vi "Arm State Controller.vi"() -> ()   [LabVIEW 2020]
uses:
  <vilib>/Rock Robotics/WPI/ThirdParty/REV Robotics/REVLib/Typedef/Spark MAX Control Type.ctl
panel:
  out "Completed Arm State":T1(ring)
  in  "Last Manual Shoulder State":dbl
  in  "Last Manual Elbow State":dbl
  in  "Target Arm State":T1(ring)
  in  "Previous Arm State":T2(ring)
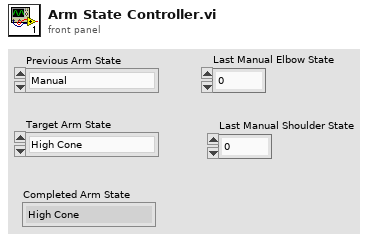
[diagram p1: front panel]
types:
  T1 = enum16{"High Cone", "Manual", "High Cube", "Mid Cone", "Mid Cube", "Intake", "Cube Handoff", "Cone Handoff", "Stow"}
  T2 = enum16{"Manual", "High Cone", "High Cube", "Mid Cone", "Mid Cube", "Intake", "Cube Handoff", "Cone Handoff", "Stow"}
  T3 = cluster{"Stow Shoulder Setpoint":dbl, "Intake Shoulder Setpoint":dbl, "Cube Handoff Shoulder Setpoint":dbl, "Cone Handoff Shoulder Setpoint":dbl, "Mid Cone Shoulder Setpoint":dbl, "Mid Cube Shoulder Setpoint":dbl, "High Cone Shoulder Setpoint":dbl, "High Cube Shoulder Setpoint":dbl}
  T4 = cluster{"Stow Elbow Setpoint":dbl, "Intake Elbow Setpoint":dbl, "Cube Handoff Elbow Setpoint":dbl, "Cone Handoff Elbow Setpoint":dbl, "Mid Cone Elbow Setpoint":dbl, "Mid Cube Elbow Setpoint":dbl, "High Cone Elbow Setpoint":dbl, "High Cube Elbow Setpoint":dbl}
  T5 = enum16{"To Manual", "From Manual", "Motion Profile", "PID Only"}
  T6 = typedef "Spark MAX Control Type.ctl" = enum16{"Percent VBus", "Voltage", "Velocity", "Position", "Smart Motion", "Current", "Smart Velocity"}
  T7 = typedef "WPI_MotorControlDeviceRef.ctl" = cluster{"DeviceStatus":errorcluster, "Type":T8, "PWM":cluster{"PWM Channel":T9, "DeadBand":T10}, "CAN":cluster{"Device Number":u8, "SetOutput VI Ref":variant, "GetOutput VI Ref":variant, "Enable VI Ref":variant, "Disable VI Ref":variant, "Data":variant}, "Invert":bool, "DIO PWM":cluster{"PWM \"Enable\" Channel":T9, "DIOChannel":T11, "PWM Rate":dbl}}
  T8 = typedef "WPI_MotorControlType.ctl" = enum16{"PWM", "CAN", "DIO PWM"}
  T9 = typedef "FPGA_DIOPWMChannel.ctl" = enum8{"PWM 0", "PWM 1", "PWM 2", "PWM 3", "PWM 4", "PWM 5", "PWM 6", "PWM 7", "PWM 8", "PWM 9", "PWM MXP 0", "PWM MXP 1", "PWM MXP 2", "PWM MXP 3", "PWM MXP 4", "PWM MXP 5", "PWM MXP 6", "PWM MXP 7", "PWM MXP 8", "PWM MXP 9", "Invalid"}
  T10 = typedef "WPI_PWMDeadband.ctl" = cluster{"Name":string, "maxPositivePwm":i32, "minPositivePwm":i32, "centerPwm":i32, "maxNegativePwm":i32, "minNegativePwm":i32, "angularRange":u16}
  T11 = typedef "FPGA_DIOChannel.ctl" = enum8{"DIO 0", "DIO 1", "DIO 2", "DIO 3", "DIO 4", "DIO 5", "DIO 6", "DIO 7", "DIO 8", "DIO 9", "DIO MXP 0", "DIO MXP 1", "DIO MXP 2", "DIO MXP 3", "DIO MXP 4", "DIO MXP 5", "DIO MXP 6", "DIO MXP 7", "DIO MXP 8", "DIO MXP 9", "DIO MXP 10", "DIO MXP 11", "DIO MXP 12", "DIO MXP 13", "DIO MXP 14", "DIO MXP 15", "SPI Port CS1", "SPI Port CS2", "SPI Port CS3", "SPI Port MISO", "SPI Port MOSI", "Invalid"}
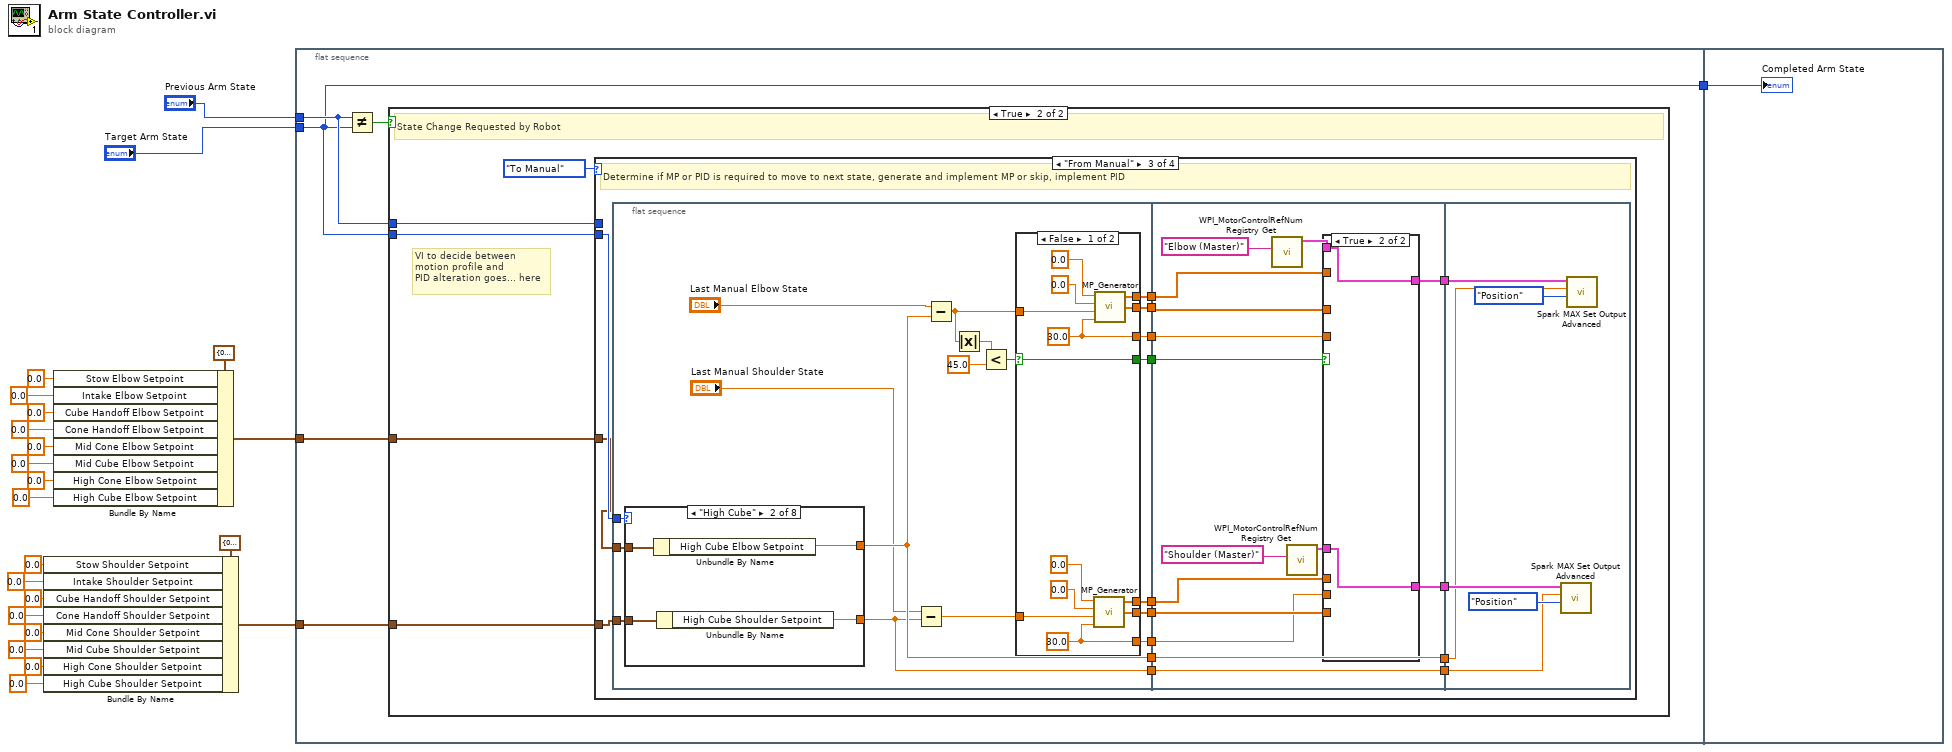
[diagram p0: block diagram]
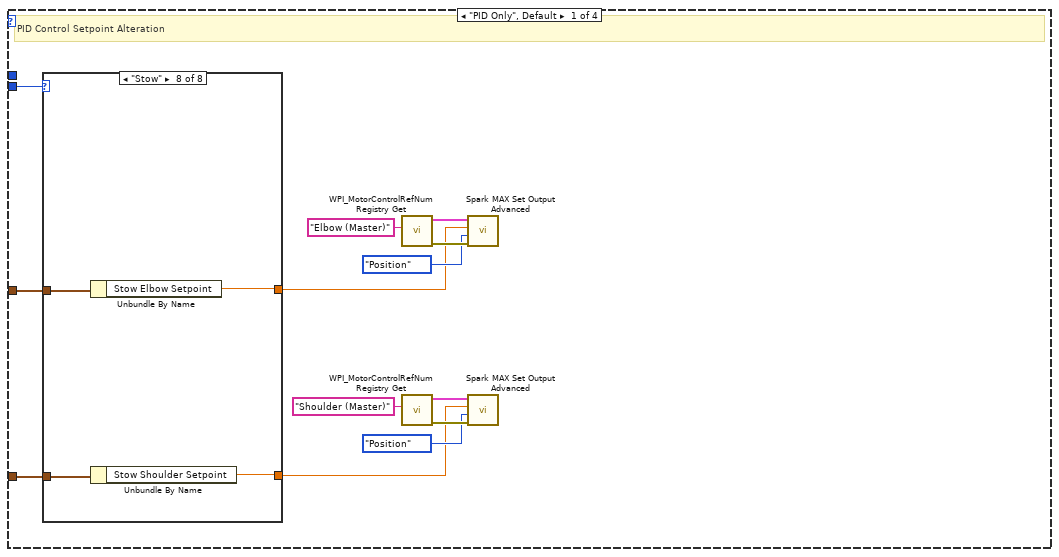
[diagram p3: hidden frame]
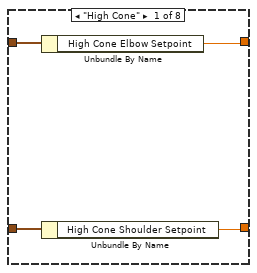
[diagram p4: hidden frame]
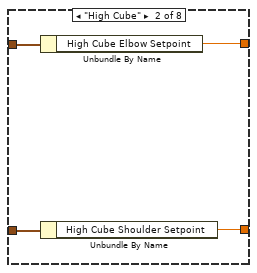
[diagram p5: hidden frame]
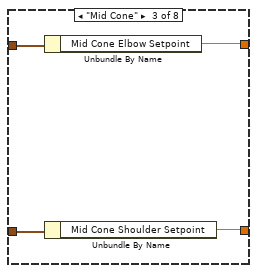
[diagram p6: hidden frame]
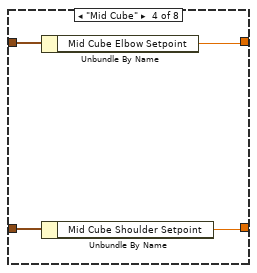
[diagram p7: hidden frame]
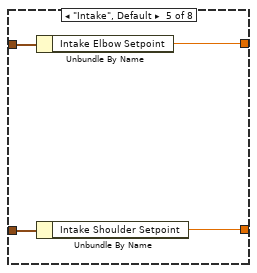
[diagram p8: hidden frame]
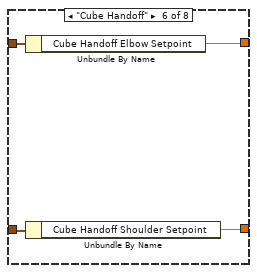
[diagram p9: hidden frame]
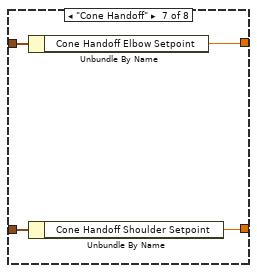
[diagram p10: hidden frame]
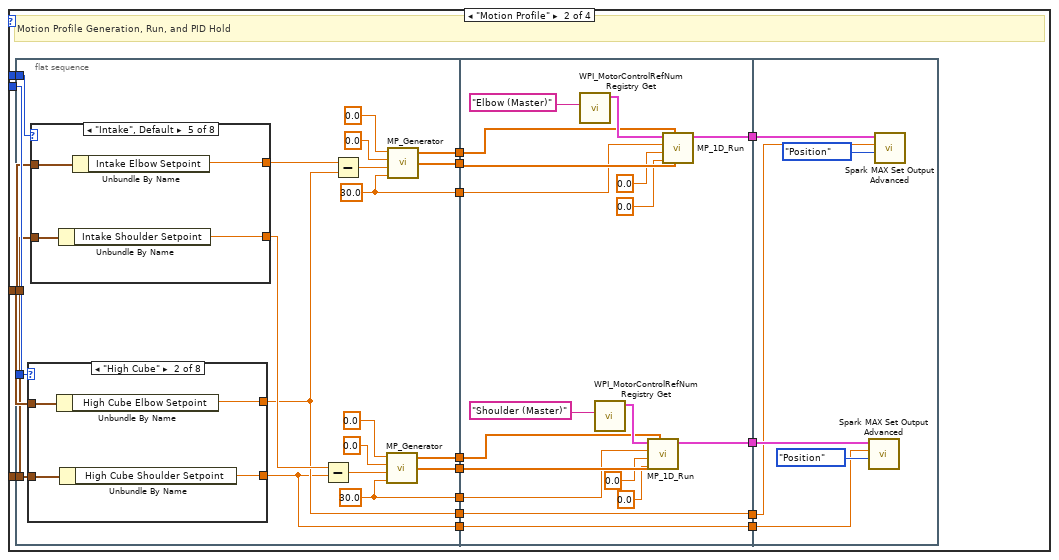
[diagram p11: hidden frame]
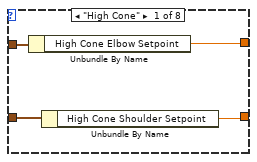
[diagram p12: hidden frame]
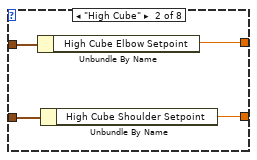
[diagram p13: hidden frame]
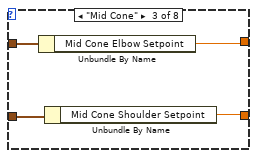
[diagram p14: hidden frame]
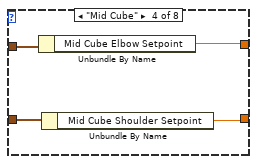
[diagram p15: hidden frame]
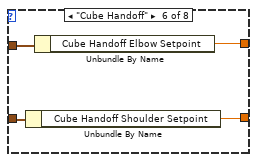
[diagram p16: hidden frame]
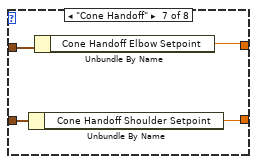
[diagram p17: hidden frame]
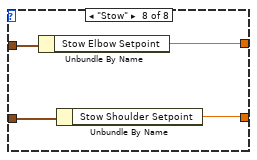
[diagram p18: hidden frame]
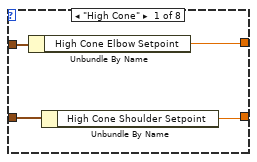
[diagram p19: hidden frame]
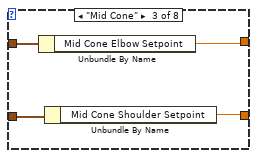
[diagram p20: hidden frame]
diagram:
  n1 = Bundle By Name(cluster=T3 {"Stow Shoulder Setpoint"=0.0, "Intake Shoulder Setpoint"=0.0, "Cube Handoff Shoulder Setpoint"=0.0, "Cone Handoff Shoulder Setpoint"=0.0, "Mid Cone Shoulder Setpoint"=0.0, "Mid Cube Shoulder Setpoint"=0.0, "High Cone Shoulder Setpoint"=0.0, "High Cube Shoulder Setpoint"=0.0}, "Stow Shoulder Setpoint"=0.0 ("Stow Elbow Setpoint"), "Intake Shoulder Setpoint"=0.0 ("Intake Elbow Setpoint"), "Cube Handoff Shoulder Setpoint"=0.0 ("Cube Handoff Elbow Setpoint"), "Cone Handoff Shoulder Setpoint"=0.0 ("Cone Handoff Elbow Setpoint"), "Mid Cone Shoulder Setpoint"=0.0 ("Mid Cone Elbow Setpoint"), "Mid Cube Shoulder Setpoint"=0.0 ("Mid Cube Elbow Setpoint"), "High Cone Shoulder Setpoint"=0.0 ("High Cone Elbow Setpoint"), "High Cube Shoulder Setpoint"=0.0 ("High Cube Elbow Setpoint")) -> (w4:T3)
  n2 = Bundle By Name(cluster=T4 {"Stow Elbow Setpoint"=0.0, "Intake Elbow Setpoint"=0.0, "Cube Handoff Elbow Setpoint"=0.0, "Cone Handoff Elbow Setpoint"=0.0, "Mid Cone Elbow Setpoint"=0.0, "Mid Cube Elbow Setpoint"=0.0, "High Cone Elbow Setpoint"=0.0, "High Cube Elbow Setpoint"=0.0}, "Stow Elbow Setpoint"=0.0, "Intake Elbow Setpoint"=0.0, "Cube Handoff Elbow Setpoint"=0.0, "Cone Handoff Elbow Setpoint"=0.0, "Mid Cone Elbow Setpoint"=0.0, "Mid Cube Elbow Setpoint"=0.0, "High Cone Elbow Setpoint"=0.0, "High Cube Elbow Setpoint"=0.0) -> (w5:T4)
  n3 = flat-sequence {
    tunnel: w5 -> [w27]
    tunnel: w4 -> [w26]
    tunnel: "Target Arm State" -> [w24]
    tunnel: "Previous Arm State" -> [w25]
    tunnel: [w24] -> w1
    tunnel: w1 -> [w324]
    frame #0 {
      n4 = Not Equal?(x=w25, y=w24) -> (x != y?=w28:bool)
      n5 = case shown="True" w28 {
        tunnel: w27 -> [_ w31]
        tunnel: w26 -> [_ w33]
        tunnel: w24 -> [_ w32]
        tunnel: w25 -> [_ w30]
        frame False {
          # "No State Change Detected"
        }
        frame True {
          # "VI to decide between\nmotion profile and \nPID alteration goes... here"
          # "State Change Requested by Robot"
          n6 = case shown="\"From Manual\"" T5."To Manual" {
            tunnel: w33 -> [w42 w92 w205 _]
            tunnel: w32 -> [w41 w94 w206 _]
            tunnel: w31 -> [w39 w93 w204 _]
            tunnel: w30 -> [_ w91 _ _]
            frame "PID Only", Default {
              # "PID Control Setpoint Alteration"
              n7 = case shown="\"Stow\"" w41 {
                tunnel: w42 -> [w48 w52 w56 w60 w66 w67 w71 w76]
                tunnel: [w47 w51 w55 w59 w65 w68 w72 w75] -> w40
                tunnel: w39 -> [w50 w54 w58 w62 w64 w70 w74 w78]
                tunnel: [w49 w53 w57 w61 w63 w69 w73 w77] -> w34
                frame "High Cone" {
                  n8 = Unbundle By Name(w50) -> ("High Cone Elbow Setpoint"=w49:dbl)
                  n9 = Unbundle By Name(w48) -> ("High Cone Shoulder Setpoint"=w47:dbl)
                }
                frame "High Cube" {
                  n10 = Unbundle By Name(w54) -> ("High Cube Elbow Setpoint"=w53:dbl)
                  n11 = Unbundle By Name(w52) -> ("High Cube Shoulder Setpoint"=w51:dbl)
                }
                frame "Mid Cone" {
                  n12 = Unbundle By Name(w58) -> ("Mid Cone Elbow Setpoint"=w57:dbl)
                  n13 = Unbundle By Name(w56) -> ("Mid Cone Shoulder Setpoint"=w55:dbl)
                }
                frame "Mid Cube" {
                  n14 = Unbundle By Name(w62) -> ("Mid Cube Elbow Setpoint"=w61:dbl)
                  n15 = Unbundle By Name(w60) -> ("Mid Cube Shoulder Setpoint"=w59:dbl)
                }
                frame "Intake", Default {
                  n16 = Unbundle By Name(w64) -> ("Intake Elbow Setpoint"=w63:dbl)
                  n17 = Unbundle By Name(w66) -> ("Intake Shoulder Setpoint"=w65:dbl)
                }
                frame "Cube Handoff" {
                  n18 = Unbundle By Name(w70) -> ("Cube Handoff Elbow Setpoint"=w69:dbl)
                  n19 = Unbundle By Name(w67) -> ("Cube Handoff Shoulder Setpoint"=w68:dbl)
                }
                frame "Cone Handoff" {
                  n20 = Unbundle By Name(w74) -> ("Cone Handoff Elbow Setpoint"=w73:dbl)
                  n21 = Unbundle By Name(w71) -> ("Cone Handoff Shoulder Setpoint"=w72:dbl)
                }
                frame "Stow" {
                  n22 = Unbundle By Name(w78) -> ("Stow Elbow Setpoint"=w77:dbl)
                  n23 = Unbundle By Name(w76) -> ("Stow Shoulder Setpoint"=w75:dbl)
                }
              }
              n24 = call <vilib>:"WPI_MotorControlRefNum Registry Get.vi"("refnum name"="Elbow (Master)") -> ("error out"=w36:errorcluster, "MotorControlDevRef"=w37:T7)  [unwired: 9 in]
              n25 = call <vilib>:"WPI_MotorControlRefNum Registry Get.vi"("refnum name"="Shoulder (Master)") -> ("error out"=w44:errorcluster, "MotorControlDevRef"=w45:T7)  [unwired: 9 in]
              n26 = call <vilib>:"Spark MAX Set Output Advanced.vi"("error in (no error)"=w36, "Control Mode"=Spark_MAX_Control_Type."Position", "Setpoint"=w34, "MotorControlDevRef"=w37) -> ()  [unwired: 6 in, 2 out]
              n27 = call <vilib>:"Spark MAX Set Output Advanced.vi"("error in (no error)"=w44, "Control Mode"=Spark_MAX_Control_Type."Position", "Setpoint"=w40, "MotorControlDevRef"=w45) -> ()  [unwired: 6 in, 2 out]
            }
            frame "Motion Profile" {
              # "Motion Profile Generation, Run, and PID Hold"
              n28 = flat-sequence {
                tunnel: w94 -> [w114]
                tunnel: w93 -> [w113]
                tunnel: w92 -> [w112]
                tunnel: w91 -> [w111]
                tunnel: [w106] -> w90
                tunnel: [w105] -> w89
                tunnel: [w100] -> w88
                tunnel: [w99] -> w87
                tunnel: [w98] -> w83
                tunnel: [w97] -> w82
                tunnel: [w96] -> w80
                tunnel: [w95] -> w79
                tunnel: w90 -> [w190]
                tunnel: w89 -> [w189]
                tunnel: w88 -> [w183]
                tunnel: w87 -> [w182]
                tunnel: [w185] -> w86
                tunnel: [w192] -> w85
                tunnel: [w194] -> w84
                tunnel: w83 -> [w194]
                tunnel: w82 -> [w193]
                tunnel: [w193] -> w81
                tunnel: w80 -> [w188]
                tunnel: w79 -> [w181]
                tunnel: w86 -> [w199]
                tunnel: w85 -> [w202]
                tunnel: w84 -> [w198]
                tunnel: w81 -> [w197]
                frame #0 {
                  w95 = 30.0 ("Time Resolution (ms)")
                  w96 = 30.0 ("Time Resolution (ms)")
                  n29 = case shown="\"High Cube\"" w114 {
                    tunnel: w112 -> [w148 w152 w156 w160 w166 w167 w171 w176]
                    tunnel: [w147 w151 w155 w159 w165 w168 w172 w175] -> w97
                    tunnel: w113 -> [w150 w154 w158 w162 w164 w170 w174 w178]
                    tunnel: [w149 w153 w157 w161 w163 w169 w173 w177] -> w98
                    frame "High Cone" {
                      n30 = Unbundle By Name(w150) -> ("High Cone Elbow Setpoint"=w149:dbl)
                      n31 = Unbundle By Name(w148) -> ("High Cone Shoulder Setpoint"=w147:dbl)
                    }
                    frame "High Cube" {
                      n32 = Unbundle By Name(w154) -> ("High Cube Elbow Setpoint"=w153:dbl)
                      n33 = Unbundle By Name(w152) -> ("High Cube Shoulder Setpoint"=w151:dbl)
                    }
                    frame "Mid Cone" {
                      n34 = Unbundle By Name(w158) -> ("Mid Cone Elbow Setpoint"=w157:dbl)
                      n35 = Unbundle By Name(w156) -> ("Mid Cone Shoulder Setpoint"=w155:dbl)
                    }
                    frame "Mid Cube" {
                      n36 = Unbundle By Name(w162) -> ("Mid Cube Elbow Setpoint"=w161:dbl)
                      n37 = Unbundle By Name(w160) -> ("Mid Cube Shoulder Setpoint"=w159:dbl)
                    }
                    frame "Intake", Default {
                      n38 = Unbundle By Name(w166) -> ("Intake Shoulder Setpoint"=w165:dbl)
                      n39 = Unbundle By Name(w164) -> ("Intake Elbow Setpoint"=w163:dbl)
                    }
                    frame "Cube Handoff" {
                      n40 = Unbundle By Name(w167) -> ("Cube Handoff Shoulder Setpoint"=w168:dbl)
                      n41 = Unbundle By Name(w170) -> ("Cube Handoff Elbow Setpoint"=w169:dbl)
                    }
                    frame "Cone Handoff" {
                      n42 = Unbundle By Name(w171) -> ("Cone Handoff Shoulder Setpoint"=w172:dbl)
                      n43 = Unbundle By Name(w174) -> ("Cone Handoff Elbow Setpoint"=w173:dbl)
                    }
                    frame "Stow" {
                      n44 = Unbundle By Name(w178) -> ("Stow Elbow Setpoint"=w177:dbl)
                      n45 = Unbundle By Name(w176) -> ("Stow Shoulder Setpoint"=w175:dbl)
                    }
                  }
                  n46 = case shown="\"Intake\", Default" w111 {
                    tunnel: w112 -> [w116 w120 w124 w128 w134 w135 w139 w144]
                    tunnel: [w115 w119 w123 w127 w133 w136 w140 w143] -> w104
                    tunnel: w113 -> [w118 w122 w126 w130 w132 w138 w142 w146]
                    tunnel: [w117 w121 w125 w129 w131 w137 w141 w145] -> w110
                    frame "High Cone" {
                      n47 = Unbundle By Name(w118) -> ("High Cone Elbow Setpoint"=w117:dbl)
                      n48 = Unbundle By Name(w116) -> ("High Cone Shoulder Setpoint"=w115:dbl)
                    }
                    frame "High Cube" {
                      n49 = Unbundle By Name(w122) -> ("High Cube Elbow Setpoint"=w121:dbl)
                      n50 = Unbundle By Name(w120) -> ("High Cube Shoulder Setpoint"=w119:dbl)
                    }
                    frame "Mid Cone" {
                      n51 = Unbundle By Name(w126) -> ("Mid Cone Elbow Setpoint"=w125:dbl)
                      n52 = Unbundle By Name(w124) -> ("Mid Cone Shoulder Setpoint"=w123:dbl)
                    }
                    frame "Mid Cube" {
                      n53 = Unbundle By Name(w130) -> ("Mid Cube Elbow Setpoint"=w129:dbl)
                      n54 = Unbundle By Name(w128) -> ("Mid Cube Shoulder Setpoint"=w127:dbl)
                    }
                    frame "Intake", Default {
                      n55 = Unbundle By Name(w134) -> ("Intake Shoulder Setpoint"=w133:dbl)
                      n56 = Unbundle By Name(w132) -> ("Intake Elbow Setpoint"=w131:dbl)
                    }
                    frame "Cube Handoff" {
                      n57 = Unbundle By Name(w135) -> ("Cube Handoff Shoulder Setpoint"=w136:dbl)
                      n58 = Unbundle By Name(w138) -> ("Cube Handoff Elbow Setpoint"=w137:dbl)
                    }
                    frame "Cone Handoff" {
                      n59 = Unbundle By Name(w139) -> ("Cone Handoff Shoulder Setpoint"=w140:dbl)
                      n60 = Unbundle By Name(w142) -> ("Cone Handoff Elbow Setpoint"=w141:dbl)
                    }
                    frame "Stow" {
                      n61 = Unbundle By Name(w146) -> ("Stow Elbow Setpoint"=w145:dbl)
                      n62 = Unbundle By Name(w144) -> ("Stow Shoulder Setpoint"=w143:dbl)
                    }
                  }
                  n63 = Subtract(x=w104, y=w97) -> (x-y=w101:dbl)
                  n64 = Subtract(x=w110, y=w98) -> (x-y=w109:dbl)
                  n65 = call "MP_Generator.vi"("Time Resolution (ms)"=w95, "Goal (deg)"=w101, "Maximum Acceleration (deg/s^2)"=0.0, "Maximum Velocity (deg/s)"=0.0) -> ("Timestamp (s)"=w99:dbl[], "Velocity (deg/s)"=w100:dbl[])  [unwired: 1 out]
                  n66 = call "MP_Generator.vi"("Time Resolution (ms)"=w96, "Goal (deg)"=w109, "Maximum Acceleration (deg/s^2)"=0.0, "Maximum Velocity (deg/s)"=0.0) -> ("Timestamp (s)"=w105:dbl[], "Velocity (deg/s)"=w106:dbl[])  [unwired: 1 out]
                }
                frame #1 {
                  n67 = call <vilib>:"WPI_MotorControlRefNum Registry Get.vi"("refnum name"="Elbow (Master)") -> ("MotorControlDevRef"=w191:T7)  [unwired: 9 in, 1 out]
                  n68 = call <vilib>:"WPI_MotorControlRefNum Registry Get.vi"("refnum name"="Shoulder (Master)") -> ("MotorControlDevRef"=w184:T7)  [unwired: 9 in, 1 out]
                  n69 = call "MP_1D_Run.vi"("Time Index"=w182, "Velocity"=w183, "Max Velocity"=0.0, "Max Acceleration"=0.0, "Time Resolution (ms)"=w181, "MotorControlDeviceRef"=w184) -> ("MotorControlDevRef"=w185:T7)  [unwired: 5 in]
                  n70 = call "MP_1D_Run.vi"("Time Index"=w189, "Velocity"=w190, "Max Velocity"=0.0, "Max Acceleration"=0.0, "Time Resolution (ms)"=w188, "MotorControlDeviceRef"=w191) -> ("MotorControlDevRef"=w192:T7)  [unwired: 5 in]
                }
                frame #2 {
                  n71 = call <vilib>:"Spark MAX Set Output Advanced.vi"("Control Mode"=Spark_MAX_Control_Type."Position", "Setpoint"=w197, "MotorControlDevRef"=w199) -> ()  [unwired: 7 in, 2 out]
                  n72 = call <vilib>:"Spark MAX Set Output Advanced.vi"("Control Mode"=Spark_MAX_Control_Type."Position", "Setpoint"=w198, "MotorControlDevRef"=w202) -> ()  [unwired: 7 in, 2 out]
                }
              }
            }
            frame "From Manual" {
              # "Determine if MP or PID is required to move to next state, generate and implement MP or skip, implement PID"
              n73 = flat-sequence {
                tunnel: w205 -> [w237]
                tunnel: [w236] -> w218
                tunnel: [w235] -> w217
                tunnel: [w234] -> w216
                tunnel: [w233] -> w215
                tunnel: [w232] -> w214
                tunnel: [w227] -> w213
                tunnel: [w231] -> w212
                tunnel: [w230] -> w211
                tunnel: w206 -> [w229]
                tunnel: w204 -> [w228]
                tunnel: [w219] -> w203
                tunnel: w218 -> [w295]
                tunnel: w217 -> [w294]
                tunnel: w216 -> [w290]
                tunnel: w215 -> [w289]
                tunnel: [w292] -> w210
                tunnel: [w297] -> w209
                tunnel: [w299] -> w208
                tunnel: w214 -> [w299]
                tunnel: w213 -> [w298]
                tunnel: [w298] -> w207
                tunnel: w212 -> [w293]
                tunnel: w211 -> [w288]
                tunnel: w203 -> [w287]
                tunnel: w210 -> [w320]
                tunnel: w209 -> [w323]
                tunnel: w208 -> [w319]
                tunnel: w207 -> [w318]
                frame #0 {
                  n74 = case shown="\"High Cube\"" w229 {
                    tunnel: w237 -> [w256 w260 w264 w268 w274 w275 w279 w284]
                    tunnel: [w255 w259 w263 w267 w273 w276 w280 w283] -> w227
                    tunnel: w228 -> [w258 w262 w266 w270 w272 w278 w282 w286]
                    tunnel: [w257 w261 w265 w269 w271 w277 w281 w285] -> w232
                    frame "High Cone" {
                      n75 = Unbundle By Name(w258) -> ("High Cone Elbow Setpoint"=w257:dbl)
                      n76 = Unbundle By Name(w256) -> ("High Cone Shoulder Setpoint"=w255:dbl)
                    }
                    frame "High Cube" {
                      n77 = Unbundle By Name(w262) -> ("High Cube Elbow Setpoint"=w261:dbl)
                      n78 = Unbundle By Name(w260) -> ("High Cube Shoulder Setpoint"=w259:dbl)
                    }
                    frame "Mid Cone" {
                      n79 = Unbundle By Name(w266) -> ("Mid Cone Elbow Setpoint"=w265:dbl)
                      n80 = Unbundle By Name(w264) -> ("Mid Cone Shoulder Setpoint"=w263:dbl)
                    }
                    frame "Mid Cube" {
                      n81 = Unbundle By Name(w270) -> ("Mid Cube Elbow Setpoint"=w269:dbl)
                      n82 = Unbundle By Name(w268) -> ("Mid Cube Shoulder Setpoint"=w267:dbl)
                    }
                    frame "Intake", Default {
                      n83 = Unbundle By Name(w274) -> ("Intake Shoulder Setpoint"=w273:dbl)
                      n84 = Unbundle By Name(w272) -> ("Intake Elbow Setpoint"=w271:dbl)
                    }
                    frame "Cube Handoff" {
                      n85 = Unbundle By Name(w275) -> ("Cube Handoff Shoulder Setpoint"=w276:dbl)
                      n86 = Unbundle By Name(w278) -> ("Cube Handoff Elbow Setpoint"=w277:dbl)
                    }
                    frame "Cone Handoff" {
                      n87 = Unbundle By Name(w279) -> ("Cone Handoff Shoulder Setpoint"=w280:dbl)
                      n88 = Unbundle By Name(w282) -> ("Cone Handoff Elbow Setpoint"=w281:dbl)
                    }
                    frame "Stow" {
                      n89 = Unbundle By Name(w286) -> ("Stow Elbow Setpoint"=w285:dbl)
                      n90 = Unbundle By Name(w284) -> ("Stow Shoulder Setpoint"=w283:dbl)
                    }
                  }
                  n91 = Subtract(x="Last Manual Shoulder State", y=w227) -> (x-y=w220:dbl)
                  n92 = Subtract(x="Last Manual Elbow State", y=w232) -> (x-y=w222:dbl)
                  n93 = Absolute Value(x=w222) -> (abs(x)=w223:dbl)
                  n94 = Less?(x=w223, y=45.0) -> (x < y?=w221:bool)
                  n95 = case shown="False" w221 {
                    selector: w221 -> [w238 w251]
                    tunnel: [w248 w254] -> w236
                    tunnel: [w247 w254] -> w235
                    tunnel: [w244 w254] -> w234
                    tunnel: [w243 w254] -> w233
                    tunnel: [w242 0.0] -> w231
                    tunnel: [w241 0.0] -> w230
                    tunnel: w222 -> [w240 _]
                    tunnel: w220 -> [w239 _]
                    tunnel: [w238 w251] -> w219
                    frame False {
                      w241 = 30.0 ("Time Resolution (ms)")
                      w242 = 30.0 ("Time Resolution (ms)")
                      n96 = call "MP_Generator.vi"("Time Resolution (ms)"=w241, "Goal (deg)"=w239, "Maximum Acceleration (deg/s^2)"=0.0, "Maximum Velocity (deg/s)"=0.0) -> ("Timestamp (s)"=w243:dbl[], "Velocity (deg/s)"=w244:dbl[])  [unwired: 1 out]
                      n97 = call "MP_Generator.vi"("Time Resolution (ms)"=w242, "Goal (deg)"=w240, "Maximum Acceleration (deg/s^2)"=0.0, "Maximum Velocity (deg/s)"=0.0) -> ("Timestamp (s)"=w247:dbl[], "Velocity (deg/s)"=w248:dbl[])  [unwired: 1 out]
                    }
                    frame True {
                      w254 = dbl[] []
                    }
                  }
                }
                frame #1 {
                  n98 = call <vilib>:"WPI_MotorControlRefNum Registry Get.vi"("refnum name"="Elbow (Master)") -> ("MotorControlDevRef"=w296:T7)  [unwired: 9 in, 1 out]
                  n99 = call <vilib>:"WPI_MotorControlRefNum Registry Get.vi"("refnum name"="Shoulder (Master)") -> ("MotorControlDevRef"=w291:T7)  [unwired: 9 in, 1 out]
                  n100 = case shown="True" w287 {
                    tunnel: [w315 w317] -> w297
                    tunnel: w296 -> [w314 w317]
                    tunnel: w295 -> [w313 _]
                    tunnel: w294 -> [w312 _]
                    tunnel: w293 -> [w311 _]
                    tunnel: [w308 w316] -> w292
                    tunnel: w291 -> [w307 w316]
                    tunnel: w290 -> [w306 _]
                    tunnel: w289 -> [w305 _]
                    tunnel: w288 -> [w304 _]
                    frame False {
                      n101 = call "MP_1D_Run.vi"("Time Index"=w305, "Velocity"=w306, "Max Velocity"=0.0, "Max Acceleration"=0.0, "Time Resolution (ms)"=w304, "MotorControlDeviceRef"=w307) -> ("MotorControlDevRef"=w308:T7)  [unwired: 5 in]
                      n102 = call "MP_1D_Run.vi"("Time Index"=w312, "Velocity"=w313, "Max Velocity"=0.0, "Max Acceleration"=0.0, "Time Resolution (ms)"=w311, "MotorControlDeviceRef"=w314) -> ("MotorControlDevRef"=w315:T7)  [unwired: 5 in]
                    }
                    frame True {
                    }
                  }
                }
                frame #2 {
                  n103 = call <vilib>:"Spark MAX Set Output Advanced.vi"("Control Mode"=Spark_MAX_Control_Type."Position", "Setpoint"=w318, "MotorControlDevRef"=w320) -> ()  [unwired: 7 in, 2 out]
                  n104 = call <vilib>:"Spark MAX Set Output Advanced.vi"("Control Mode"=Spark_MAX_Control_Type."Position", "Setpoint"=w319, "MotorControlDevRef"=w323) -> ()  [unwired: 7 in, 2 out]
                }
              }
            }
            frame "To Manual" {
              # "Shouldn't do much of anything here. Manual control will be tackled by a separate VI.\nThis is mostly a catch to make sure this VI does not take action when the state changes to manual."
            }
          }
        }
      }
    }
    frame #1 {
      "Completed Arm State" <- w324
    }
  }
